vi "AutotoolRegions.vi"(5 "XRef":refnum<vi>, 6 "State In":T1={"Input Type"=variant(dbl 0.0), "Width"=0, "Typedef Name"="", "Value Type"=variant, "Selection"=0, "Options"=[], "Selections"=[], "Display Selections"=[], "Element Names"=[], "Typedef Name Width"=0, "Display Selection Width"=[], "Code Generated"=FALSE}) -> (2 "Regions":T7)   [LabVIEW 2015, in "Read-Write-Signals.xnode"]
doc: "This ability VI is called by LabVIEW to determine which tool to use when hovering over an xnode in edit mode, if autotool is turned on. The Bounds of each region is a rectangular region of the xnode in coordinates relative to the top left corner of the xnode. Tool is the autotool that should be used when the user hovers over the particular region of the xnode.\n \n LabVIEW will sort the Regions by Priority so that lower priority regions are tried first in determining what tool to use.\n \n This VI cannot override autotool behavior on grow handles and terminal whiskers of xnodes.\n \n LabVIEW may cache the Regions array and can also call this VI if the Regions array is not currently cached. To force LabVIEW to call this VI and update its autotool regions, use the Reply of \"UpdateAutotoolRegions\".\n\nDefault behavior: None.\n\nThis ability does not provide UI and OS messages are not handled."
uses:
  Read-Write-Signals.xnode
  <vilib>/XNodeSupport/XNodeAutotoolRegions.ctl
  <vilib>/XNodeSupport/XNodeAutotoolRegion.ctl
  <vilib>/XNodeSupport/XNodeRect32.ctl
  <vilib>/XNodeSupport/XNodeInt.ctl
  <vilib>/XNodeSupport/XNodeTools.ctl
  State.ctl
  Read-Write-Signals Item.ctl
  Read-Write-Signals Sub Item.ctl
  Read-Write-Signals Sub Item Type.ctl
  Read-Write-Signals Selection.ctl
  Read-Write-Signals Display Selection.ctl
  <vilib>/XNodeSupport/NI_XNodeSupport.lvlib
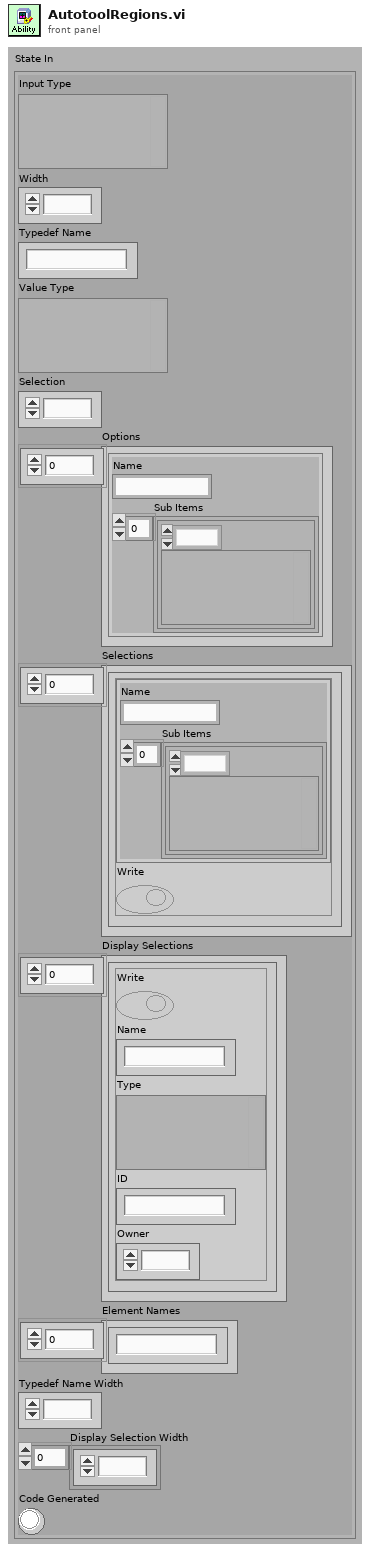
[diagram p1: front panel]
types:
  T1 = typedef "Read-Write-Signals.xnode/State.ctl" = cluster{"Input Type":variant, "Width":i32, "Typedef Name":string, "Value Type":variant, "Selection":i32, "Options":T2[], "Selections":T5[], "Display Selections":T6[], "Element Names":string[], "Typedef Name Width":i32, "Display Selection Width":i32[], "Code Generated":bool}
  T2 = typedef "Read-Write-Signals Item.ctl" = cluster{"Name":string, "Sub Items":T3[]}
  T3 = typedef "Read-Write-Signals Sub Item.ctl" = cluster{"Type":T4, "Value":variant}
  T4 = typedef "Read-Write-Signals Sub Item Type.ctl" = enum8{"Cluster Element", "Array Element", "Subarray"}
  T5 = typedef "Read-Write-Signals Selection.ctl" = cluster{"Item":T2, "Write":bool}
  T6 = typedef "Read-Write-Signals Display Selection.ctl" = cluster{"Write":bool, "Name":string, "Type":variant, "ID":string, "Owner":i32}
  T7 = typedef "NI_XNodeSupport.lvlib/XNodeAutotoolRegions.ctl" = T8[]
  T8 = typedef "NI_XNodeSupport.lvlib/XNodeAutotoolRegion.ctl" = cluster{"Bounds":T9, "Autotool":T11}
  T9 = typedef "NI_XNodeSupport.lvlib/XNodeRect32.ctl" = cluster{"Left":T10, "Top":T10, "Right":T10, "Bottom":T10}
  T10 = typedef "NI_XNodeSupport.lvlib/XNodeInt.ctl" = i32
  T11 = typedef "NI_XNodeSupport.lvlib/XNodeTools.ctl" = enum32{"Operating Tool", "Placement Tool", "Labelling Tool", "Wiring Tool", "Scroll Tool", "Breakpoint Tool", "Probe Tool", "Auto Tool"}
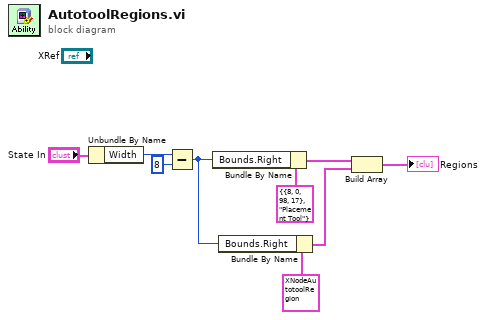
[diagram p0: block diagram]
diagram:
  n1 = Unbundle By Name("State In") -> ("Width"=w2:i32)
  n2 = Subtract(x=w2, y=8) -> (x-y=w4:i32)
  n3 = Bundle By Name(cluster=T8 {"Bounds"={"Left"=8, "Top"=0, "Right"=98, "Bottom"=17}, "Autotool"=enum."Placement Tool"} ("Autotool Region"), "Bounds.Right"=w4) -> (w6:T8)
  n4 = Bundle By Name(cluster=T8 {"Bounds"={"Left"=8, "Top"=18, "Right"=90, "Bottom"=1000}, "Autotool"=enum."Operating Tool"} ("Autotool Region"), "Bounds.Right"=w4) -> (w5:T8)
  n5 = Build Array(w6, w5) -> (→"Regions":T8[])
